vi "NavbalLabVIEW(15-5-28.vi"() -> ()   [LabVIEW 2012] (continued)
              n343 = Index Array(array=w4186, index=1) -> (element=w4183:i32)
              n344 = Insert Into Array(array=w4184, index (dim 1)=w4183, new element=w4182) -> (w4178:dbl[][][])  [unwired: 2 in]
              n345 = Array Size(array=w4178) -> (size(s)=w4180:i32[])
              n346 = Index Array(array=w4180, index=1) -> (element=w4179:i32)
              n347 = Insert Into Array(array=w4178, index (dim 1)=w4179, new element=w4177) -> (w4176:dbl[][][])  [unwired: 2 in]
            }
            frame "LA Class" {
              n348 = Array Size(array=w4200) -> (size(s)=w4201:i32[])
              n349 = Array Size(array=w4203) -> (size(s)=w4206:i32[])
              n350 = Index Array(array=w4201, index=1) -> (element=w4199:i32)
              n351 = Index Array(array=w4206, index=1) -> (element=w4204:i32)
              n352 = Insert Into Array(array=w4200, index (dim 1)=w4199, new element=w4198) -> (w4193:dbl[][][])  [unwired: 2 in]
              n353 = Insert Into Array(array=w4203, index (dim 1)=w4204, new element=w4207) -> (w4194:dbl[][][])  [unwired: 2 in]
              n354 = Array Size(array=w4194) -> (size(s)=w4197:i32[])
              n355 = Index Array(array=w4197, index=1) -> (element=w4195:i32)
              n356 = Insert Into Array(array=w4194, index (dim 1)=w4195, new element=w4193) -> (w4192:dbl[][][])  [unwired: 2 in]
            }
            frame "Ohio Class" {
              n357 = Array Size(array=w4216) -> (size(s)=w4217:i32[])
              n358 = Array Size(array=w4219) -> (size(s)=w4222:i32[])
              n359 = Index Array(array=w4217, index=1) -> (element=w4215:i32)
              n360 = Index Array(array=w4222, index=1) -> (element=w4220:i32)
              n361 = Insert Into Array(array=w4219, index (dim 1)=w4220, new element=w4223) -> (w4210:dbl[][][])  [unwired: 2 in]
              n362 = Insert Into Array(array=w4216, index (dim 1)=w4215, new element=w4214) -> (w4209:dbl[][][])  [unwired: 2 in]
              n363 = Array Size(array=w4210) -> (size(s)=w4213:i32[])
              n364 = Index Array(array=w4213, index=1) -> (element=w4211:i32)
              n365 = Insert Into Array(array=w4210, index (dim 1)=w4211, new element=w4209) -> (w4208:dbl[][][])  [unwired: 2 in]
            }
          }
          n366 = Array Size(array=w3330) -> (size(s)=w3436:i32[])
          n367 = Array Size(array=w3333) -> (size(s)=w3427:i32[])
          n368 = Array Size(array=w3332) -> (size(s)=w3425:i32[])
          n369 = Array Size(array=w3331) -> (size(s)=w3420:i32[])
          n370 = Index Array(array=w3436, index=0) -> (element=w3418:i32)
          n371 = Index Array(array=w3427, index=0) -> (element=w3426:i32)
          n372 = Index Array(array=w3425, index=0) -> (element=w3423:i32)
          n373 = Index Array(array=w3420, index=0) -> (element=w3419:i32)
          n374 = Greater?(x=w3418, y=700) -> (0:w3429:bool)
          n375 = Or(x="Mark Current", y=w3366) -> (x .or. y?=w3367:bool)
          n376 = case shown="True" "Averaging" {
            tunnel: [10 "Number of Averages"] -> w3416
            frame False {
            }
            frame True {
            }
          }
          n377 = case shown="\"Simulated Signals Ohio\"" w3369 {
            tunnel: [w4382 w4431 w4480] -> w3480
            tunnel: [w4386 w4435 w4484] -> w3478
            tunnel: [w4384 w4433 w4482] -> w3523
            tunnel: [w4373 w4428 w4477] -> w3328
            tunnel: [w4385 w4434 w4483] -> w3407
            tunnel: [w4383 w4432 w4481] -> w3406
            tunnel: [w4381 w4430 w4479] -> w3456
            tunnel: [w4380 w4429 w4478] -> w3532
            tunnel: w3530 -> [w4387 w4436 w4485]
            tunnel: w3416 -> [w4374 w4422 w4471]
            frame "Simulated Signals Ohio" {
              # "Ensure that buffer is full before processing"
              # ">>  data out from buffer  >>"
              n378 = local read "Number of Samples"() -> (w4388:i32)
              n379 = call "Convert to Dynamic Data11"("Array"=bool[] [FALSE, FALSE, FALSE, FALSE, FALSE, FALSE, FALSE, FALSE, FALSE, FALSE, TRUE, FALSE, FALSE, FALSE, FALSE, FALSE, FALSE, FALSE, FALSE, FALSE]) -> ("Dynamic Data Type"=w4376:dynamicdata)  [unwired: 3 in]
              n380 = call-poly <userlib>:"Circular Buffer.vi"("Buffer Size"=w4387, "Read Size"=w4388, "Operation"=Circular_Buffer_Operations."Read (most recent)") -> ("Data Out"=w4375:waveform(dbl)[])  [unwired: 5 in, 3 out]
              n381 = call "Select Tach Port2"("Selector Input"=w4376, "Signals"=w4375) -> ("Signal Out"=w4380:dynamicdata)  [unwired: 8 in, 1 out]
              n382 = call "Convert from Dynamic Data49"("Dynamic Data Type"=w4375) -> ("Array"=w4391:dbl[][])  [unwired: 3 in]
              n383 = call "Convert to Dynamic Data10"("Array"=bool[] [TRUE, FALSE, FALSE, FALSE, FALSE, FALSE, FALSE, FALSE, FALSE, FALSE, FALSE, FALSE, FALSE, FALSE, FALSE, FALSE, FALSE, FALSE, FALSE, FALSE]) -> ("Dynamic Data Type"=w4378:dynamicdata)  [unwired: 3 in]
              n384 = Array Size(array=w4391) -> (size(s)=w4394:i32[])
              n385 = call "Select Tach Stbd3"("Selector Input"=w4378, "Signals"=w4375) -> ("Signal Out"=w4373:dynamicdata)  [unwired: 8 in, 1 out]
              n386 = Equal?(x=w4394, y=w4388) -> (x = y?=w4392:bool[])
              n387 = Index Array(array=w4392, index=1) -> (element=w4389:bool)
              n388 = case shown="True" w4389 {
                tunnel: w4375 -> [_ w4414]
                tunnel: [w4395 w4407] -> w4386
                tunnel: [w4397 w4404] -> w4385
                tunnel: [w4395 w4406] -> w4384
                tunnel: [w4395 w4405] -> w4382
                tunnel: [w4397 w4401] -> w4383
                tunnel: [w4397 w4402] -> w4381
                tunnel: w4374 -> [_ w4400]
                frame False {
                  w4395 = cluster{"x0":dbl, "dx":dbl, "magnitude":dbl[]}[] [] ("spectra")
                  n389 = local read "DAQ Start"() -> (w4396:bool)
                  n390 = case shown="True" w4396 {
                    frame False {
                      n391 = property on="DAQ Start" class="Bool (strict)"("BoolText.Text"="DAQ START" ("Boolean Text.Text")) -> ()  [unwired: 2 in, 2 out]
                    }
                    frame True {
                      n392 = property on="DAQ Start" class="Bool (strict)"("BoolText.Text"="Buffering..." ("Boolean Text.Text")) -> ()  [unwired: 2 in, 2 out]
                    }
                  }
                  n393 = local read "Default Stbd Graph"() -> (w4397:dynamicdata)
                }
                frame True {
                  # "convert to VdB"
                  # "convert to VdB"
                  # "convert to VdB"
                  n394 = local read "DAQ Start"() -> (w4403:bool)
                  n395 = case shown="True" w4403 {
                    frame False {
                    }
                    frame True {
                      n396 = property on="DAQ Start" class="Bool (strict)"("BoolText.Text"="DAQ STOP" ("Boolean Text.Text")) -> ()  [unwired: 2 in, 2 out]
                    }
                  }
                  n397 = call "Convert to Dynamic Data3"("Array"=bool[] [FALSE, FALSE, FALSE, FALSE, FALSE, FALSE, FALSE, FALSE, FALSE, FALSE, TRUE, TRUE, TRUE, TRUE, TRUE, TRUE, TRUE, TRUE, TRUE, TRUE]) -> ("Dynamic Data Type"=w4415:dynamicdata)  [unwired: 3 in]
                  n398 = call "Select Port"("Selector Input"=w4415, "Signals"=w4414) -> ("Signal Out"=w4401:dynamicdata)  [unwired: 8 in, 1 out]
                  n399 = call "Convert to Dynamic Data2"("Array"=bool[] [TRUE, TRUE, TRUE, TRUE, TRUE, TRUE, TRUE, TRUE, TRUE, TRUE, FALSE, FALSE, FALSE, FALSE, FALSE, FALSE, FALSE, FALSE, FALSE, FALSE]) -> ("Dynamic Data Type"=w4419:dynamicdata)  [unwired: 3 in]
                  n400 = call "Select Stbd"("Selector Input"=w4419, "Signals"=w4414) -> ("Signal Out"=w4404:dynamicdata)  [unwired: 8 in, 1 out]
                  n401 = call "Convert to Dynamic Data4"("Array"=bool[] [FALSE, FALSE, FALSE, FALSE, FALSE, FALSE, FALSE, FALSE, FALSE, FALSE, FALSE, FALSE, FALSE, FALSE, FALSE, FALSE, FALSE, FALSE, FALSE, FALSE, TRUE, TRUE, TRUE, TRUE, TRUE, TRUE, TRUE, TRUE, TRUE, TRUE, TRUE, TRUE]) -> ("Dynamic Data Type"=w4416:dynamicdata)  [unwired: 3 in]
                  n402 = call "Select Corner"("Selector Input"=w4416, "Signals"=w4414) -> ("Signal Out"=w4402:dynamicdata)  [unwired: 8 in, 1 out]
                  n403 = call-poly <vilib>:"SVL Set dB Reference.vi"("dB reference [EU]"=3.937e-07, "scaled signals in [EU]"=w4404) -> ("scaled signals out [EU]"=w4412:waveform(dbl)[])  [unwired: 8 in, 1 out]
                  n404 = call-poly <vilib>:"SVL Set dB Reference.vi"("dB reference [EU]"=3.937e-07, "scaled signals in [EU]"=w4402) -> ("scaled signals out [EU]"=w4408:waveform(dbl)[])  [unwired: 8 in, 1 out]
                  n405 = call-poly <vilib>:"SVL Set dB Reference.vi"("dB reference [EU]"=3.937e-07, "scaled signals in [EU]"=w4401) -> ("scaled signals out [EU]"=w4410:waveform(dbl)[])  [unwired: 8 in, 1 out]
                  n406 = call "Power Spectrum3"("input signals"=w4410, "number of averages"=w4400) -> ("spectra"=w4406:cluster{"x0":dbl, "dx":dbl, "magnitude":dbl[]}[])  [unwired: 12 in, 5 out]
                  n407 = call "Power Spectrum6"("input signals"=w4408, "number of averages"=w4400) -> ("spectra"=w4405:cluster{"x0":dbl, "dx":dbl, "magnitude":dbl[]}[])  [unwired: 12 in, 5 out]
                  n408 = call "Power Spectrum2"("input signals"=w4412, "number of averages"=w4400) -> ("spectra"=w4407:cluster{"x0":dbl, "dx":dbl, "magnitude":dbl[]}[])  [unwired: 12 in, 5 out]
                }
              }
            }
            frame "LA Class" {
              # "Ensure that buffer is full before processing"
              # ">>  data out from buffer  >>"
              n409 = local read "Number of Samples"() -> (w4437:i32)
              n410 = call "Convert to Dynamic Data19"("Array"=bool[] [FALSE, FALSE, FALSE, FALSE, FALSE, FALSE, FALSE, FALSE, FALSE, FALSE, FALSE, FALSE, FALSE, FALSE, FALSE, FALSE, FALSE, FALSE, FALSE, FALSE, FALSE, FALSE, FALSE, FALSE, FALSE, TRUE]) -> ("Dynamic Data Type"=w4424:dynamicdata)  [unwired: 3 in]
              n411 = call-poly <userlib>:"Circular Buffer.vi"("Buffer Size"=w4436, "Read Size"=w4437, "Operation"=Circular_Buffer_Operations."Read (most recent)") -> ("Data Out"=w4423:waveform(dbl)[])  [unwired: 5 in, 3 out]
              n412 = call "Select Tach Port4"("Selector Input"=w4424, "Signals"=w4423) -> ("Signal Out"=w4429:dynamicdata)  [unwired: 8 in, 1 out]
              n413 = call "Convert from Dynamic Data5"("Dynamic Data Type"=w4423) -> ("Array"=w4440:dbl[][])  [unwired: 3 in]
              n414 = call "Convert to Dynamic Data18"("Array"=bool[] [TRUE, FALSE, FALSE, FALSE, FALSE, FALSE, FALSE, FALSE, FALSE, FALSE, FALSE, FALSE, FALSE, FALSE, FALSE, FALSE, FALSE, FALSE, FALSE, FALSE]) -> ("Dynamic Data Type"=w4426:dynamicdata)  [unwired: 3 in]
              n415 = Array Size(array=w4440) -> (size(s)=w4443:i32[])
              n416 = call "Select Tach Stbd2"("Selector Input"=w4426, "Signals"=w4423) -> ("Signal Out"=w4428:dynamicdata)  [unwired: 8 in, 1 out]
              n417 = Equal?(x=w4443, y=w4437) -> (x = y?=w4441:bool[])
              n418 = Index Array(array=w4441, index=1) -> (element=w4438:bool)
              n419 = case shown="False" w4438 {
                tunnel: w4423 -> [_ w4466]
                tunnel: [w4444 w4459] -> w4435
                tunnel: [w4446 w4456] -> w4434
                tunnel: [w4444 w4458] -> w4433
                tunnel: [w4444 w4457] -> w4431
                tunnel: [w4446 w4453] -> w4432
                tunnel: [w4446 w4454] -> w4430
                tunnel: w4422 -> [_ w4452]
                frame False {
                  w4444 = cluster{"x0":dbl, "dx":dbl, "magnitude":dbl[]}[] [] ("spectra")
                  n420 = local read "DAQ Start"() -> (w4445:bool)
                  n421 = case shown="True" w4445 {
                    frame False {
                      n422 = property on="DAQ Start" class="Bool (strict)"("BoolText.Text"="DAQ START" ("Boolean Text.Text")) -> ()  [unwired: 2 in, 2 out]
                    }
                    frame True {
                      n423 = property on="DAQ Start" class="Bool (strict)"("BoolText.Text"="Buffering..." ("Boolean Text.Text")) -> ()  [unwired: 2 in, 2 out]
                    }
                  }
                  n424 = local read "Default Stbd Graph"() -> (w4446:dynamicdata)
                }
                frame True {
                  # "convert to VdB"
                  # "convert to VdB"
                  # "convert to VdB"
                  n425 = local read "DAQ Start"() -> (w4455:bool)
                  n426 = case shown="True" w4455 {
                    frame False {
                    }
                    frame True {
                      n427 = property on="DAQ Start" class="Bool (strict)"("BoolText.Text"="DAQ STOP" ("Boolean Text.Text")) -> ()  [unwired: 2 in, 2 out]
                    }
                  }
                  n428 = call "Convert to Dynamic Data16"("Array"=bool[] [FALSE, FALSE, FALSE, FALSE, FALSE, FALSE, FALSE, FALSE, FALSE, FALSE, FALSE, FALSE, FALSE, FALSE, FALSE, FALSE, FALSE, FALSE, FALSE, FALSE, FALSE, FALSE, FALSE, FALSE, FALSE, TRUE, TRUE, TRUE, TRUE, TRUE, TRUE, TRUE, TRUE, TRUE, TRUE, TRUE, TRUE, TRUE]) -> ("Dynamic Data Type"=w4467:dynamicdata)  [unwired: 3 in]
                  n429 = call "Select Port3"("Selector Input"=w4467, "Signals"=w4466) -> ("Signal Out"=w4453:dynamicdata)  [unwired: 8 in, 1 out]
                  n430 = call "Convert to Dynamic Data15"("Array"=bool[] [TRUE, FALSE, FALSE, FALSE, FALSE, FALSE, FALSE, FALSE, FALSE, FALSE, FALSE, FALSE, FALSE, TRUE, TRUE, TRUE, TRUE, TRUE, TRUE, TRUE, TRUE, TRUE, TRUE, TRUE, TRUE, FALSE, FALSE, FALSE, FALSE, FALSE, FALSE, FALSE, FALSE, FALSE, FALSE, FALSE, FALSE, FALSE]) -> ("Dynamic Data Type"=w4469:dynamicdata)  [unwired: 3 in]
                  n431 = call "Select Stbd4"("Selector Input"=w4469, "Signals"=w4466) -> ("Signal Out"=w4456:dynamicdata)  [unwired: 8 in, 1 out]
                  n432 = call "Convert to Dynamic Data17"("Array"=bool[] [FALSE, TRUE, TRUE, TRUE, TRUE, TRUE, TRUE, TRUE, TRUE, TRUE, TRUE, TRUE, TRUE, FALSE, FALSE, FALSE, FALSE, FALSE, FALSE, FALSE, FALSE, FALSE, FALSE, FALSE, FALSE, FALSE, FALSE, FALSE, FALSE, FALSE, FALSE, FALSE, FALSE, FALSE, FALSE, FALSE, FALSE, FALSE]) -> ("Dynamic Data Type"=w4468:dynamicdata)  [unwired: 3 in]
                  n433 = call "Select Corner4"("Selector Input"=w4468, "Signals"=w4466) -> ("Signal Out"=w4454:dynamicdata)  [unwired: 8 in, 1 out]
                  n434 = call-poly <vilib>:"SVL Set dB Reference.vi"("dB reference [EU]"=3.937e-07, "scaled signals in [EU]"=w4456) -> ("scaled signals out [EU]"=w4464:waveform(dbl)[])  [unwired: 8 in, 1 out]
                  n435 = call-poly <vilib>:"SVL Set dB Reference.vi"("dB reference [EU]"=3.937e-07, "scaled signals in [EU]"=w4454) -> ("scaled signals out [EU]"=w4460:waveform(dbl)[])  [unwired: 8 in, 1 out]
                  n436 = call-poly <vilib>:"SVL Set dB Reference.vi"("dB reference [EU]"=3.937e-07, "scaled signals in [EU]"=w4453) -> ("scaled signals out [EU]"=w4462:waveform(dbl)[])  [unwired: 8 in, 1 out]
                  n437 = call "Power Spectrum12"("input signals"=w4460, "number of averages"=w4452) -> ("spectra"=w4457:cluster{"x0":dbl, "dx":dbl, "magnitude":dbl[]}[])  [unwired: 12 in, 5 out]
                  n438 = call "Power Spectrum11"("input signals"=w4462, "number of averages"=w4452) -> ("spectra"=w4458:cluster{"x0":dbl, "dx":dbl, "magnitude":dbl[]}[])  [unwired: 12 in, 5 out]
                  n439 = call "Power Spectrum10"("input signals"=w4464, "number of averages"=w4452) -> ("spectra"=w4459:cluster{"x0":dbl, "dx":dbl, "magnitude":dbl[]}[])  [unwired: 12 in, 5 out]
                }
              }
            }
            frame "Ohio Class" {
              # "Ensure that buffer is full before processing"
              # ">>  data out from buffer  >>"
              n440 = local read "Number of Samples"() -> (w4486:i32)
              n441 = call "Convert to Dynamic Data24"("Array"=bool[] [FALSE, FALSE, FALSE, FALSE, FALSE, FALSE, FALSE, FALSE, FALSE, FALSE, FALSE, FALSE, FALSE, FALSE, FALSE, FALSE, FALSE, FALSE, FALSE, FALSE, FALSE, FALSE, TRUE]) -> ("Dynamic Data Type"=w4473:dynamicdata)  [unwired: 3 in]
              n442 = call-poly <userlib>:"Circular Buffer.vi"("Buffer Size"=w4485, "Read Size"=w4486, "Operation"=Circular_Buffer_Operations."Read (most recent)") -> ("Data Out"=w4472:waveform(dbl)[])  [unwired: 5 in, 3 out]
              n443 = call "Select Tach Port5"("Selector Input"=w4473, "Signals"=w4472) -> ("Signal Out"=w4478:dynamicdata)  [unwired: 8 in, 1 out]
              n444 = call "Convert from Dynamic Data6"("Dynamic Data Type"=w4472) -> ("Array"=w4489:dbl[][])  [unwired: 3 in]
              n445 = call "Convert to Dynamic Data23"("Array"=bool[] [TRUE, FALSE, FALSE, FALSE, FALSE, FALSE, FALSE, FALSE, FALSE, FALSE, FALSE, FALSE, FALSE, FALSE, FALSE, FALSE, FALSE, FALSE, FALSE, FALSE]) -> ("Dynamic Data Type"=w4475:dynamicdata)  [unwired: 3 in]
              n446 = Array Size(array=w4489) -> (size(s)=w4492:i32[])
              n447 = call "Select Tach Stbd5"("Selector Input"=w4475, "Signals"=w4472) -> ("Signal Out"=w4477:dynamicdata)  [unwired: 8 in, 1 out]
              n448 = Equal?(x=w4492, y=w4486) -> (x = y?=w4490:bool[])
              n449 = Index Array(array=w4490, index=1) -> (element=w4487:bool)
              n450 = case shown="False" w4487 {
                tunnel: w4472 -> [_ w4512]
                tunnel: [w4493 w4505] -> w4484
                tunnel: [w4495 w4502] -> w4483
                tunnel: [w4493 w4504] -> w4482
                tunnel: [w4493 w4503] -> w4480
                tunnel: [w4495 w4499] -> w4481
                tunnel: [w4495 w4500] -> w4479
                tunnel: w4471 -> [_ w4498]
                frame False {
                  w4493 = cluster{"x0":dbl, "dx":dbl, "magnitude":dbl[]}[] [] ("spectra")
                  n451 = local read "DAQ Start"() -> (w4494:bool)
                  n452 = case shown="True" w4494 {
                    frame False {
                      n453 = property on="DAQ Start" class="Bool (strict)"("BoolText.Text"="DAQ START" ("Boolean Text.Text")) -> ()  [unwired: 2 in, 2 out]
                    }
                    frame True {
                      n454 = property on="DAQ Start" class="Bool (strict)"("BoolText.Text"="Buffering..." ("Boolean Text.Text")) -> ()  [unwired: 2 in, 2 out]
                    }
                  }
                  n455 = local read "Default Stbd Graph"() -> (w4495:dynamicdata)
                }
                frame True {
                  # "convert to VdB"
                  # "convert to VdB"
                  # "convert to VdB"
                  n456 = local read "DAQ Start"() -> (w4501:bool)
                  n457 = case shown="True" w4501 {
                    frame False {
                    }
                    frame True {
                      n458 = property on="DAQ Start" class="Bool (strict)"("BoolText.Text"="DAQ STOP" ("Boolean Text.Text")) -> ()  [unwired: 2 in, 2 out]
                    }
                  }
                  n459 = call "Convert to Dynamic Data21"("Array"=bool[] [FALSE, FALSE, FALSE, FALSE, FALSE, FALSE, FALSE, FALSE, FALSE, FALSE, FALSE, FALSE, FALSE, FALSE, FALSE, FALSE, FALSE, FALSE, FALSE, FALSE, FALSE, FALSE, TRUE, TRUE, TRUE, TRUE, TRUE, TRUE, TRUE, TRUE, TRUE, TRUE]) -> ("Dynamic Data Type"=w4513:dynamicdata)  [unwired: 3 in]
                  n460 = call "Select Port5"("Selector Input"=w4513, "Signals"=w4512) -> ("Signal Out"=w4499:dynamicdata)  [unwired: 8 in, 1 out]
                  n461 = call "Convert to Dynamic Data20"("Array"=bool[] [TRUE, FALSE, FALSE, FALSE, FALSE, FALSE, FALSE, FALSE, FALSE, FALSE, FALSE, FALSE, FALSE, TRUE, TRUE, TRUE, TRUE, TRUE, TRUE, TRUE, TRUE, TRUE]) -> ("Dynamic Data Type"=w4517:dynamicdata)  [unwired: 3 in]
                  n462 = call "Select Stbd5"("Selector Input"=w4517, "Signals"=w4512) -> ("Signal Out"=w4502:dynamicdata)  [unwired: 8 in, 1 out]
                  n463 = call "Convert to Dynamic Data22"("Array"=bool[] [FALSE, TRUE, TRUE, TRUE, TRUE, TRUE, TRUE, TRUE, TRUE, TRUE, TRUE, TRUE, TRUE, FALSE, FALSE, FALSE, FALSE, FALSE, FALSE, FALSE, FALSE, FALSE, FALSE, FALSE, FALSE, FALSE, FALSE, FALSE, FALSE, FALSE, FALSE, FALSE]) -> ("Dynamic Data Type"=w4514:dynamicdata)  [unwired: 3 in]
                  n464 = call "Select Corner5"("Selector Input"=w4514, "Signals"=w4512) -> ("Signal Out"=w4500:dynamicdata)  [unwired: 8 in, 1 out]
                  n465 = call-poly <vilib>:"SVL Set dB Reference.vi"("dB reference [EU]"=3.937e-07, "scaled signals in [EU]"=w4502) -> ("scaled signals out [EU]"=w4510:waveform(dbl)[])  [unwired: 8 in, 1 out]
                  n466 = call-poly <vilib>:"SVL Set dB Reference.vi"("dB reference [EU]"=3.937e-07, "scaled signals in [EU]"=w4500) -> ("scaled signals out [EU]"=w4506:waveform(dbl)[])  [unwired: 8 in, 1 out]
                  n467 = call-poly <vilib>:"SVL Set dB Reference.vi"("dB reference [EU]"=3.937e-07, "scaled signals in [EU]"=w4499) -> ("scaled signals out [EU]"=w4508:waveform(dbl)[])  [unwired: 8 in, 1 out]
                  n468 = call "Power Spectrum15"("input signals"=w4506, "number of averages"=w4498) -> ("spectra"=w4503:cluster{"x0":dbl, "dx":dbl, "magnitude":dbl[]}[])  [unwired: 12 in, 5 out]
                  n469 = call "Power Spectrum13"("input signals"=w4510, "number of averages"=w4498) -> ("spectra"=w4505:cluster{"x0":dbl, "dx":dbl, "magnitude":dbl[]}[])  [unwired: 12 in, 5 out]
                  n470 = call "Power Spectrum14"("input signals"=w4508, "number of averages"=w4498) -> ("spectra"=w4504:cluster{"x0":dbl, "dx":dbl, "magnitude":dbl[]}[])  [unwired: 12 in, 5 out]
                }
              }
            }
          }
          "Default Stbd Graph" <- w3407
          "spectra" <- w3523
          n471 = call "Convert from Dynamic Data48"("Dynamic Data Type"=w3532) -> ("Array"=w3544:dbl[])  [unwired: 3 in]
          n472 = Array Max & Min(array=w3544) -> (max value=w3533:dbl)  [unwired: 3 out]
          n473 = Greater?(x=w3533, y=1.0) -> (0:w3542:bool)
          n474 = case shown="True" w3542 {
            tunnel: w3532 -> [_ w4362]
            tunnel: [0.0 ("detected frequency") w4359] -> w3538
            frame False {
            }
            frame True {
              n475 = call "Filter2"("Lower Cut-Off"="Port Tach Cutoff Freq", "Signal"=w4362) -> ("Filtered Signal"=w4357:dynamicdata)  [unwired: 8 in, 1 out]
              n476 = call "Power Spectrum4"("input signals"=w4357) -> ("spectra"=→"Port Tach Spectra":cluster{"x0":dbl, "dx":dbl, "magnitude":dbl[]}[])  [unwired: 13 in, 5 out]
              n477 = call-poly <vilib>:"Extract Single Tone Information.vi"("time signals in"=w4357) -> ("detected frequencies"=w4361:dbl[])  [unwired: 5 in, 5 out]
              n478 = Index Array(array=w4361, index=0) -> (element=w4359:dbl)
            }
          }
          "Frequency (Hz) 2" <- w3538
          n479 = Multiply(x=w3538, y=60.0) -> (x*y=→"Frequency (RPM) 2":dbl)
          n480 = In Range and Coerce(upper limit=60.6, x=w3538, lower limit=60.4) -> (In Range?=w3535:bool)  [unwired: 1 out]
          n481 = case shown="True" w3535 {
            tunnel: [u32 16752008 u32 5308226] -> w3534
            frame False {
            }
            frame True {
            }
          }
          n482 = property on="Frequency (Hz) 2" class="DigNum (strict)"("NumText.BGColor"=w3534) -> ()  [unwired: 2 in, 2 out]
          n483 = property on="Frequency (RPM) 2" class="DigNum (strict)"("NumText.BGColor"=w3534) -> ()  [unwired: 2 in, 2 out]
          n484 = call "Convert from Dynamic Data47"("Dynamic Data Type"=w3328) -> ("Array"=w3554:dbl[])  [unwired: 3 in]
          n485 = Array Max & Min(array=w3554) -> (max value=w3551:dbl)  [unwired: 3 out]
          n486 = Greater?(x=w3551, y=1.0) -> (0:w3552:bool)
          n487 = case shown="True" w3552 {
            tunnel: w3328 -> [_ w4370]
            tunnel: [0.0 ("detected frequency") w4369] -> w3537
            frame False {
            }
            frame True {
              n488 = call "Filter"("Lower Cut-Off"="Stbd Tach Cutoff Freq", "Signal"=w4370) -> ("Filtered Signal"=w4367:dynamicdata)  [unwired: 8 in, 1 out]
              n489 = call-poly <vilib>:"Extract Single Tone Information.vi"("time signals in"=w4367) -> ("detected frequencies"=w4371:dbl[])  [unwired: 5 in, 5 out]
              n490 = Index Array(array=w4371, index=0) -> (element=w4369:dbl)
              n491 = call "Power Spectrum"("input signals"=w4367) -> ("spectra"=→"Starboard Tach Spectra":cluster{"x0":dbl, "dx":dbl, "magnitude":dbl[]}[])  [unwired: 13 in, 5 out]
            }
          }
          "Frequency (Hz) 1" <- w3537
          n492 = Multiply(x=w3537, y=60.0) -> (x*y=→"Frequency (RPM) 1":dbl)
          n493 = In Range and Coerce(upper limit=59.6, x=w3537, lower limit=59.4) -> (In Range?=w3549:bool)  [unwired: 1 out]
          n494 = case shown="True" w3549 {
            tunnel: [u32 16752008 u32 5308226] -> w3545
            frame False {
            }
            frame True {
            }
          }
          n495 = property on="Frequency (Hz) 1" class="DigNum (strict)"("NumText.BGColor"=w3545) -> ()  [unwired: 2 in, 2 out]
          n496 = property on="Frequency (RPM) 1" class="DigNum (strict)"("NumText.BGColor"=w3545) -> ()  [unwired: 2 in, 2 out]
          n497 = case shown="True" w3367 {
            frame False {
            }
            frame True {
              n498 = local read "time string"() -> (→"Marker Time":string)
              n499 = local read "Mils/Sec-Phase(CORNERS-Stbd)"() -> (w4242:sgl[][])
              n500 = local read "Mils/Sec-Phase(CORNERS-Port)"() -> (w4245:sgl[][])
              n501 = local read "Mils/Sec-Phase(STBD)"() -> (w4244:dbl[][])
              n502 = local read "Mils/Sec-Phase(PORT)"() -> (w4243:sgl[][])
              n503 = Array Size(array=w4242) -> (size(s)=w4241:i32[])
              n504 = Index Array(array=w4241, index=0) -> (element=w4239:i32)
              n505 = Insert Into Array(array=w4242, index (row)=w4239, new element #1=w4245, new element #2=w4244, new element #3=w4243) -> (w4238:sgl[][])  [unwired: 1 in]
              n506 = local read "Marker Mag"() -> (w4234:sgl[][])
              n507 = local read "Marker Phase"() -> (w4227:sgl[][])
              n508 = Index Array "Mag"(array=w4238, index (col)=0 ("disabled index (col)")) -> (element=w4235:sgl[])  [unwired: 1 in]
              n509 = Index Array "Phase"(array=w4238, index (col)=1 ("disabled index (col)")) -> (element=w4226:sgl[])  [unwired: 1 in]
              n510 = Array Size(array=w4234) -> (size(s)=w4233:i32[])
              n511 = Array Size(array=w4227) -> (size(s)=w4228:i32[])
              n512 = Index Array(array=w4233, index=1) -> (element=w4231:i32)
              n513 = Insert Into Array(array=w4234, index (col)=w4231, new element=w4235) -> (→"Marker Mag":sgl[][])  [unwired: 1 in]
              n514 = Index Array(array=w4228, index=1) -> (element=w4225:i32)
              n515 = Insert Into Array(array=w4227, index (col)=w4225, new element=w4226) -> (→"Marker Phase":sgl[][])  [unwired: 1 in]
            }
          }
          n516 = case shown="True" w3429 {
            tunnel: [w3940 w3944] -> w3434
            tunnel: w3333 -> [w3940 w3957]
            tunnel: [w3939 w3943] -> w3433
            tunnel: w3332 -> [w3939 w3955]
            tunnel: [w3938 w3942] -> w3432
            tunnel: w3331 -> [w3938 w3950]
            tunnel: [w3937 w3941] -> w3431
            tunnel: w3330 -> [w3937 w3948]
            tunnel: w3426 -> [_ w3956]
            tunnel: w3423 -> [_ w3954]
            tunnel: 600 ("y") -> [_ w3945]
            tunnel: w3419 -> [_ w3951]
            tunnel: w3418 -> [_ w3947]
            frame False {
            }
            frame True {
              n517 = Subtract(x=w3956, y=w3945) -> (x-y=w3953:i32)
              n518 = Subtract(x=w3954, y=w3945) -> (x-y=w3952:i32)
              n519 = Subtract(x=w3951, y=w3945) -> (x-y=w3949:i32)
              n520 = Subtract(x=w3947, y=w3945) -> (x-y=w3946:i32)
              n521 = Delete From Array(array=w3957, length=w3953, index (dim 0)=w3945) -> (array with subset deleted=w3944:dbl[][][])  [unwired: 2 in, 1 out]
              n522 = Delete From Array(array=w3955, length=w3952, index (dim 0)=w3945) -> (array with subset deleted=w3943:dbl[][][])  [unwired: 2 in, 1 out]
              n523 = Delete From Array(array=w3950, length=w3949, index (dim 0)=w3945) -> (array with subset deleted=w3942:dbl[][][])  [unwired: 2 in, 1 out]
              n524 = Delete From Array(array=w3948, length=w3946, index (dim 0)=w3945) -> (array with subset deleted=w3941:dbl[][][])  [unwired: 2 in, 1 out]
            }
          }
          n525 = Array Subset(array=w3334, index (dim 0)=0 ("index"), length (dim 0)=600 ("length"), index (dim 1)="DAQ Listbox", length (dim 1)=1 ("length"), index (dim 2)=0 ("index"), length (dim 2)=2 ("length")) -> (w3610:dbl[][][])
          n526 = Array Subset(array=w3334, index (dim 0)=0 ("index"), length (dim 0)=1 ("length"), index (dim 1)="DAQ Listbox", length (dim 1)=1 ("length"), index (dim 2)=0 ("index"), length (dim 2)=2 ("length")) -> (w3595:dbl[][][])
          n527 = Reshape Array(w3610, 600 ("dimension size"), 2 ("dimension size")) -> (w3572:dbl[][])
          n528 = Reshape Array(w3595, 1 ("dimension size"), 2 ("dimension size")) -> (w3582:dbl[][])
          n529 = Index Array(array=w3582, index (col)=0 ("disabled index (col)")) -> (element=w3584:dbl[])  [unwired: 1 in]
          n530 = Index Array(array=w3582, index (col)=1 ("disabled index (col)")) -> (element=w3581:dbl[])  [unwired: 1 in]
          n531 = Array Subset(array=w3572, index (row)=0 ("index"), length (row)=600 ("length"), index (col)=0 ("index"), length (col)=1 ("length")) -> (w3573:dbl[][])
          n532 = Array Subset(array=w3572, index (row)=0 ("index"), length (row)=600 ("length"), index (col)=1 ("index"), length (col)=1 ("length")) -> (w3597:dbl[][])
          n533 = Reshape Array(w3584, 1 ("dimension size")) -> (w3585:dbl[])
          n534 = Reshape Array(w3581, 1 ("dimension size")) -> (w3591:dbl[])
          n535 = Index Array(array=w3585, index=0) -> (element=w3579:dbl)
          n536 = Index Array(array=w3591, index=0) -> (element=w3616:dbl)
          n537 = Reshape Array(w3597, 600 ("dimension size")) -> (w3576:dbl[])
          n538 = Reshape Array(w3573, 600 ("dimension size")) -> (w3580:dbl[])
          n539 = Insert Into Array(array=w3580, index=0, new element=w3579) -> (→"mag":dbl[])
          n540 = Insert Into Array(array=w3576, index=0, new element=w3616) -> (→"phase":dbl[])
          n541 = property on="Tab 3" class="TabCtl (strict)"() -> ("Visible"=w3443:bool)  [unwired: 2 in, 2 out]
          n542 = property on="Tab 3" class="TabCtl (strict)"() -> ("Value"=w3446:T9)  [unwired: 2 in, 2 out]
          n543 = Equal?(x=w3446, y=T19."Step 6: Polar Plots") -> (x = y?=w3444:bool)
          n544 = And(x=w3444, y=w3443) -> (x .and. y?=w3442:bool)
          n545 = case shown="True" w3442 {
            frame False {
            }
            frame True {
              w3989 = 0 ("index")
              w4002 = T21."Application Font" ("desired font(Application)")
              w4004 = cluster{"width":i16, "height":i16} {"width"=575, "height"=575} ("dimensions (w,h)")
              # "Find the max magnitude to be plotted,\nand adjust the scaling of all plots"
              # "Add Corresponding Prediction measurement to Polar plot"
              # "Add Corresponding Baseline measurement to Polar plot"
              # "Polar Plot"
              n546 = local read "Marker Phase"() -> (w3970:sgl[][])
              n547 = local read "Pred plot"() -> (w3958:dbl[][])
              n548 = local read "Marker Mag"() -> (w3963:sgl[][])
              n549 = Array Size(array=w3963) -> (size(s)=w3966:i32[])
              n550 = local read "Ref Pt Plot"() -> (w3976:sgl[][])
              n551 = Index Array(array=w3966, index=1) -> (element=w3964:i32)
              n552 = local read "DAQ Listbox"() -> (w3969:i32)
              n553 = Index Array(array=w3958, index (col)=1 ("disabled index (col)")) -> (element=w3959:dbl[])  [unwired: 1 in]
              n554 = Index Array(array=w3958, index (col)=0 ("disabled index (col)")) -> (element=w3960:dbl[])  [unwired: 1 in]
              n555 = for {
                N: w3964 -> [_]
                tunnel: [w4013] -> w3968
                tunnel: [w4015] -> w3967 mode=indexing
                tunnel: w3969 -> [w4014]
                tunnel: w3970 -> [w4008]
                tunnel: w3963 -> [w4007]
                i -> [w4011]
                n556 = Index Array(array=w4007, index (row)=w4014) -> (element=w4013:sgl[])  [unwired: 1 in]
                n557 = Index Array(array=w4008, index (row)=w4014) -> (element=w4012:sgl[])  [unwired: 1 in]
                n558 = Index Array(array=w4012, index=w4011) -> (element=w4009:sgl)
                n559 = Index Array(array=w4013, index=w4011) -> (element=w4010:sgl)
                n560 = Bundle(w4010, w4009) -> (w4015:cluster{sgl, sgl})  [unwired: 1 in]
              }
              n561 = Index Array(array=w3976, index (col)=0 ("disabled index (col)")) -> (element=w3978:sgl[])  [unwired: 1 in]
              n562 = Index Array(array=w3976, index (col)=1 ("disabled index (col)")) -> (element=w3975:sgl[])  [unwired: 1 in]
              n563 = Index Array(array=w3959, index=w3969) -> (element=w3991:dbl)
              n564 = Index Array(array=w3960, index=w3969) -> (element=w3988:dbl)
              n565 = for {
                N: 600 -> [_]
                tunnel: [w4020] -> w4003 mode=indexing
                i -> [w4021]
                n566 = local read "phase"() -> (w4016:dbl[])
                n567 = local read "mag"() -> (w4017:dbl[])
                n568 = Index Array(array=w4017, index=w4021) -> (element=w4019:dbl)
                n569 = Index Array(array=w4016, index=w4021) -> (element=w4018:dbl)
                n570 = Bundle("mag. (Vpeak)"=w4019, "mag. (Vpeak)"=w4018) -> (w4020:cluster{"mag. (Vpeak)":dbl, "mag. (Vpeak)":dbl})  [unwired: 1 in]
              }
              n571 = local read "mag"() -> (w3994:dbl[])
              n572 = Bundle("Real Matrix Element"=w3988, "Real Matrix Element"=w3991) -> (w3983:T22)  [unwired: 1 in]
              n573 = Index Array(array=w3978, index=w3969) -> (element=w3993:sgl)
              n574 = Index Array(array=w3975, index=w3969) -> (element=w3997:sgl)
              n575 = Insert Into Array(array=w3994, index=w3989, new element #1=w3993, new element #2=0 ("new element/subarray"), new element #3=w3968) -> (w3990:dbl[])
              n576 = Bundle(w3993, w3997) -> (w3996:cluster{sgl, sgl})  [unwired: 1 in]
              n577 = Initialize Array(w3983, 1 ("dimension size")) -> (w3982:T23)
              n578 = Initialize Array(w3996, 1 ("dimension size")) -> (w3992:cluster{sgl, sgl}[])
              n579 = Insert Into Array(array=w3990, index=w3989, new element=w3988) -> (w3987:dbl[])
              n580 = Array Max & Min(array=w3987) -> (max value=w3980:dbl)  [unwired: 3 out]
              n581 = Divide(x=w3980, y=0.9) -> (x/y=w3971:dbl)
              n582 = property on="maximum" class="DigNum (strict)"("Val(Sgnl)"=w3971) -> ()  [unwired: 2 in, 2 out]
              n583 = call <vilib>:"Polar Plot(points&line).vi"("polar attributes"="polar attributes", "desired font(Application)"=w4002, "dimensions (w,h)"=w4004, "data array [mag, phase (deg)]"=w4003) -> ("new picture"=w3999:picture)  [unwired: 7 in]
              n584 = property on="maximum" class="DigNum (strict)"("Val(Sgnl)"=w3971) -> ()  [unwired: 2 in, 2 out]
              n585 = property on="maximum" class="DigNum (strict)"("Val(Sgnl)"=w3971) -> ()  [unwired: 2 in, 2 out]
              n586 = property on="maximum" class="DigNum (strict)"("Val(Sgnl)"=w3971) -> ()  [unwired: 2 in, 2 out]
              n587 = feedback #1() -> (w3998:picture)  [unwired: 1 in]
              n588 = call <vilib>:"Polar Plot(points&line).vi"("polar attributes"="polar attributes Prediction", "desired font(Application)"=w4002, "dimensions (w,h)"=w4004, "data array [mag, phase (deg)]"=w3982, "picture"=w3998) -> ("new picture"=w3986:picture)  [unwired: 6 in]
              n589 = call <vilib>:"Polar Plot(points&line).vi"("polar attributes"="polar attributes Start Point", "desired font(Application)"=w4002, "dimensions (w,h)"=w4004, "data array [mag, phase (deg)]"=w3992, "picture"=w3986) -> ("new picture"=w3973:picture)  [unwired: 6 in]
              n590 = call <vilib>:"Polar Plot(points&line).vi"("polar attributes"="polar attributes Marker", "desired font(Application)"=w4002, "dimensions (w,h)"=w4004, "data array [mag, phase (deg)]"=w3967, "picture"=w3973) -> ("new picture"=→"Polar Plot Picture":picture)  [unwired: 6 in]
              n591 = feedback-in #1(w3999) -> ()
            }
          }
          n592 = local read "Ship Class"() -> (w3555:T4)
          n593 = local read "Frequency (Hz) 1"() -> (w3556:dbl)
          n594 = case shown="\"LA Class\"" w3555 {
            tunnel: w3407 -> [w4860 w4875 w4876]
            tunnel: [w4846 w4861 w4878] -> w3457
            tunnel: [w4859 w4874 w4877] -> w3477
            frame "LA Class" {
              n595 = Split Signals(w4860) -> (w4859:dynamicdata, w4858:dynamicdata, w4857:dynamicdata, w4856:dynamicdata, w4855:dynamicdata, w4854:dynamicdata, w4853:dynamicdata, w4852:dynamicdata, w4851:dynamicdata, w4850:dynamicdata, w4849:dynamicdata, w4848:dynamicdata, w4847:dynamicdata)  [unwired: 13 in]
              n596 = Merge Signals(w4858, w4857, w4856, w4855, w4854, w4853, w4852, w4851, w4850, w4849, w4848, w4847) -> (w4846:dynamicdata)
            }
            frame "Ohio Class" {
              n597 = Split Signals(w4875) -> (w4874:dynamicdata, w4873:dynamicdata, w4872:dynamicdata, w4871:dynamicdata, w4870:dynamicdata, w4869:dynamicdata, w4868:dynamicdata, w4867:dynamicdata, w4866:dynamicdata, w4865:dynamicdata, w4864:dynamicdata, w4863:dynamicdata, w4862:dynamicdata)  [unwired: 13 in]
              n598 = Merge Signals(w4873, w4872, w4871, w4870, w4869, w4868, w4867, w4866, w4865, w4864, w4863, w4862) -> (w4861:dynamicdata)
            }
            frame "Simulated Signals Ohio" {
              n599 = Split Signals(w4876) -> (w4877:dynamicdata, w4879:dynamicdata, w4880:dynamicdata, w4881:dynamicdata, w4882:dynamicdata, w4883:dynamicdata, w4884:dynamicdata, w4885:dynamicdata, w4886:dynamicdata, w4887:dynamicdata)  [unwired: 10 in]
              n600 = Merge Signals(w4879, w4880, w4881, w4882, w4883, w4884, w4885, w4886, w4887) -> (w4878:dynamicdata)
            }
          }
          n601 = local read "Sample Frequency (Hz)"() -> (w3528:i32)
          n602 = local read "Sample Frequency (Hz)"() -> (w3529:i32)
          n603 = local read "Sample Frequency (Hz)"() -> (w3527:i32)
          n604 = local read "Sample Frequency (Hz)"() -> (w3482:i32)
          n605 = case shown="\"Simulated Signals Ohio\"" w3555 {
            tunnel: w3406 -> [w4807 w4830 w4845]
            tunnel: [w4806 w4816 w4831] -> w3665
            tunnel: [w4805 w4829 w4844] -> w3666
            frame "Simulated Signals Ohio" {
              n606 = Split Signals(w4807) -> (w4805:dynamicdata, w4808:dynamicdata, w4809:dynamicdata, w4810:dynamicdata, w4811:dynamicdata, w4812:dynamicdata, w4813:dynamicdata, w4814:dynamicdata, w4815:dynamicdata, w4804:dynamicdata)  [unwired: 10 in]
              n607 = Merge Signals(w4808, w4809, w4810, w4811, w4812, w4813, w4814, w4815, w4804) -> (w4806:dynamicdata)
            }
            frame "LA Class" {
              n608 = Split Signals(w4830) -> (w4829:dynamicdata, w4828:dynamicdata, w4827:dynamicdata, w4826:dynamicdata, w4825:dynamicdata, w4824:dynamicdata, w4823:dynamicdata, w4822:dynamicdata, w4821:dynamicdata, w4820:dynamicdata, w4819:dynamicdata, w4818:dynamicdata, w4817:dynamicdata)  [unwired: 13 in]
              n609 = Merge Signals(w4828, w4827, w4826, w4825, w4824, w4823, w4822, w4821, w4820, w4819, w4818, w4817) -> (w4816:dynamicdata)
            }
            frame "Ohio Class" {
              n610 = Split Signals(w4845) -> (w4844:dynamicdata, w4843:dynamicdata, w4842:dynamicdata, w4841:dynamicdata, w4840:dynamicdata, w4839:dynamicdata, w4838:dynamicdata, w4837:dynamicdata, w4836:dynamicdata, w4835:dynamicdata, w4834:dynamicdata, w4833:dynamicdata, w4832:dynamicdata)  [unwired: 13 in]
              n611 = Merge Signals(w4843, w4842, w4841, w4840, w4839, w4838, w4837, w4836, w4835, w4834, w4833, w4832) -> (w4831:dynamicdata)
            }
          }
          n612 = local read "Frequency (Hz) 2"() -> (w3557:dbl)
          n613 = local read "Frequency (Hz) 1"() -> (w3643:dbl)
          n614 = local read "Frequency (Hz) 2"() -> (w3483:dbl)
          n615 = Array Size(array=w3523) -> (size(s)=w3520:i32)
          n616 = Array Size(array=w3478) -> (size(s)=w3531:i32)
          n617 = Decrement(x=w3520) -> (x-1=w3519:i32)
          n618 = Decrement(x=w3531) -> (x-1=w3521:i32)
          n619 = Array Size(array=w3480) -> (size(s)=w3571:i32)
          n620 = Array Size(array=w3480) -> (size(s)=w3481:i32)
          n621 = for "Phase (Degrees)" {
            N: w3519 -> [_]
            tunnel: w3406 -> [w4983]
            tunnel: [w4985] -> w3691 mode=indexing
            tunnel: w3528 -> [w4984]
            i -> [w4988]
            n622 = Add(x=1, y=w4988) -> (x+y=w4986:i32)
            n623 = call "Convert from Dynamic Data30"("Dynamic Data Type"=w4983, "Channel"=w4986) -> ("Array"=w4991:dbl[])  [unwired: 2 in]
            n624 = call "Convert from Dynamic Data31"("Dynamic Data Type"=w4983, "Channel"=0) -> ("Array"=w4989:dbl[])  [unwired: 2 in]
            n625 = Reciprocal(x=w4984) -> (1/x=w4995:dbl)
            n626 = call <vilib>:"Cross Power Spectrum.vi"("dt"=w4995, "Signal Y (V)"=w4991, "Signal X (V)"=w4989) -> ("Cross Power XY Spectrum Phase (radians)"=w4982:dbl[])  [unwired: 2 out]
            n627 = Divide(x=180, y=3.141592653589793) -> (x/y=w4992:dbl)
            n628 = Multiply(x=w4982, y=w4992) -> (x*y=w4985:dbl[])
          }
          n629 = for "Magnitude (VdB)" {
            N: w3521 -> [_]
            tunnel: w3478 -> [w5057]
            tunnel: [w5053] -> w3704 mode=indexing
            i -> [w5056]
            n630 = Add(x=1, y=w5056) -> (x+y=w5054:i32)
            n631 = Index Array(array=w5057, index=w5054) -> (element=w5058:cluster{"x0":dbl, "dx":dbl, "magnitude":dbl[]})
            n632 = Unbundle(w5058) -> ("magnitude"=w5053:dbl[])  [unwired: 2 out]
          }
          n633 = Index Array(array=w3478) -> (element=w3705:cluster{"x0":dbl, "dx":dbl, "magnitude":dbl[]})  [unwired: 1 in]
          n634 = for "Phase (Degrees)" {
            N: w3521 -> [_]
            tunnel: w3407 -> [w5095]
            tunnel: [w5091] -> w3559 mode=indexing
            tunnel: w3529 -> [w5089]
            i -> [w5093]
            n635 = Add(x=1, y=w5093) -> (x+y=w5090:i32)
            n636 = call "Convert from Dynamic Data27"("Dynamic Data Type"=w5095, "Channel"=w5090) -> ("Array"=w5097:dbl[])  [unwired: 2 in]
            n637 = call "Convert from Dynamic Data28"("Dynamic Data Type"=w5095, "Channel"=0) -> ("Array"=w5094:dbl[])  [unwired: 2 in]
            n638 = Reciprocal(x=w5089) -> (1/x=w5102:dbl)
            n639 = call <vilib>:"Cross Power Spectrum.vi"("dt"=w5102, "Signal Y (V)"=w5097, "Signal X (V)"=w5094) -> ("Cross Power XY Spectrum Phase (radians)"=w5101:dbl[])  [unwired: 2 out]
            n640 = Divide(x=180, y=3.141592653589793) -> (x/y=w5098:dbl)
            n641 = Multiply(x=w5101, y=w5098) -> (x*y=w5091:dbl[])
          }
          n642 = for "Magnitude (VdB)" {
            N: w3519 -> [_]
            tunnel: w3523 -> [w4949]
            tunnel: [w4945] -> w3689 mode=indexing
            i -> [w4948]
            n643 = Add(x=1, y=w4948) -> (x+y=w4946:i32)
            n644 = Index Array(array=w4949, index=w4946) -> (element=w4950:cluster{"x0":dbl, "dx":dbl, "magnitude":dbl[]})
            n645 = Unbundle(w4950) -> ("magnitude"=w4945:dbl[])  [unwired: 2 out]
          }
          n646 = Index Array(array=w3523) -> (element=w3690:cluster{"x0":dbl, "dx":dbl, "magnitude":dbl[]})  [unwired: 1 in]
          n647 = for "Magnitude (VdB)" {
            N: w3571 -> [_]
            tunnel: w3480 -> [w4758]
            tunnel: [w4757] -> w3662 mode=indexing
            i -> [w4756]
            n648 = Index Array(array=w4758, index=w4756) -> (element=w4759:cluster{"x0":dbl, "dx":dbl, "magnitude":dbl[]})
            n649 = Unbundle(w4759) -> ("magnitude"=w4757:dbl[])  [unwired: 2 out]
          }
          n650 = Unbundle(w3705) -> ("dx"=w3703:dbl)  [unwired: 2 out]
          "frequency resolution" <- w3703
          n651 = Index Array(array=w3480) -> (element=w3663:cluster{"x0":dbl, "dx":dbl, "magnitude":dbl[]})  [unwired: 1 in]
          n652 = for "Phase (Degrees)" {
            N: w3571 -> [_]
            tunnel: w3456 -> [w4796]
            tunnel: [w4794] -> w3664 mode=indexing
            tunnel: w3407 -> [w4792]
            tunnel: w3527 -> [w4791]
            i -> [w4793]
            n653 = call "Convert from Dynamic Data33"("Dynamic Data Type"=w4796, "Channel"=w4793) -> ("Array"=w4798:dbl[])  [unwired: 2 in]
            n654 = call "Convert from Dynamic Data34"("Dynamic Data Type"=w4792, "Channel"=0) -> ("Array"=w4795:dbl[])  [unwired: 2 in]
            n655 = Reciprocal(x=w4791) -> (1/x=w4803:dbl)
            n656 = call <vilib>:"Cross Power Spectrum.vi"("dt"=w4803, "Signal Y (V)"=w4798, "Signal X (V)"=w4795) -> ("Cross Power XY Spectrum Phase (radians)"=w4802:dbl[])  [unwired: 2 out]
            n657 = Divide(x=180, y=3.141592653589793) -> (x/y=w4799:dbl)
            n658 = Multiply(x=w4802, y=w4799) -> (x*y=w4794:dbl[])
          }
          n659 = Unbundle(w3690) -> ("dx"=w3688:dbl)  [unwired: 2 out]
          n660 = for "Magnitude (VdB)" {
            N: w3481 -> [_]
            tunnel: w3480 -> [w4307]
            tunnel: [w4306] -> w3513 mode=indexing
            i -> [w4305]
            n661 = Index Array(array=w4307, index=w4305) -> (element=w4308:cluster{"x0":dbl, "dx":dbl, "magnitude":dbl[]})
            n662 = Unbundle(w4308) -> ("magnitude"=w4306:dbl[])  [unwired: 2 out]
          }
          n663 = Index Array(array=w3480) -> (element=w3514:cluster{"x0":dbl, "dx":dbl, "magnitude":dbl[]})  [unwired: 1 in]
          n664 = for "Phase (Degrees)" {
            N: w3481 -> [_]
            tunnel: w3456 -> [w4345]
            tunnel: [w4343] -> w3515 mode=indexing
            tunnel: w3406 -> [w4341]
            tunnel: w3482 -> [w4340]
            i -> [w4342]
            n665 = call "Convert from Dynamic Data"("Dynamic Data Type"=w4345, "Channel"=w4342) -> ("Array"=w4347:dbl[])  [unwired: 2 in]
            n666 = call "Convert from Dynamic Data2"("Dynamic Data Type"=w4341, "Channel"=0) -> ("Array"=w4344:dbl[])  [unwired: 2 in]
            n667 = Reciprocal(x=w4340) -> (1/x=w4352:dbl)
            n668 = call <vilib>:"Cross Power Spectrum.vi"("dt"=w4352, "Signal Y (V)"=w4347, "Signal X (V)"=w4344) -> ("Cross Power XY Spectrum Phase (radians)"=w4351:dbl[])  [unwired: 2 out]
            n669 = Divide(x=180, y=3.141592653589793) -> (x/y=w4348:dbl)
            n670 = Multiply(x=w4351, y=w4348) -> (x*y=w4343:dbl[])
          }
          n671 = Unbundle(w3663) -> ("dx"=w3661:dbl)  [unwired: 2 out]
          "frequency (resolution) corner" <- w3661
          n672 = Unbundle(w3514) -> ("dx"=w3512:dbl)  [unwired: 2 out]
          "frequency (resolution) corners-port" <- w3512
          n673 = for "Mag (VdB)(8x)" {
            N: w3521 -> [_]
            tunnel: w3704 -> [w5039]
            tunnel: w3703 -> [w5037]
            tunnel: w3556 -> [w5035]
            tunnel: [w5034] -> w3696 mode=indexing
            i -> [w5036]
            n674 = Index Array(array=w5039, index (row)=w5036) -> (element=w5033:dbl[])  [unwired: 1 in]
            n675 = for {
              N: 8 -> [_]
              tunnel: [w5044] -> w5034 mode=indexing
              tunnel: w5033 -> [w5048]
              tunnel: w5035 -> [w5050]
              tunnel: w5037 -> [w5052]
              i -> [w5049]
              w5042 = ext 2.0  # change
              n676 = Divide(x=w5050, y=w5052) -> (x/y=w5040:dbl)
              n677 = Multiply(x=w5040, y=w5049) -> (x*y=w5051:dbl)
              n678 = Add(x=w5040, y=w5051) -> (x+y=w5046:dbl)
              n679 = Subtract(x=w5046, y=w5042) -> (x-y=w5047:ext)
              n680 = Multiply(x=w5042, y=2.0) -> (x*y=w5041:ext)
              n681 = Array Subset(array=w5048, index=w5047, length=w5041) -> (w5045:dbl[])
              n682 = Array Max & Min(array=w5045) -> (max value=w5044:dbl)  [unwired: 3 out]
            }
          }
          "Magnitude VdB Stbd" <- w3696
          n683 = for "Mag (VdB)(8x)" {
            N: w3519 -> [_]
            tunnel: w3689 -> [w4931]
            tunnel: w3688 -> [w4929]
            tunnel: w3557 -> [w4927]
            tunnel: [w4926] -> w3681 mode=indexing
            i -> [w4928]
            n684 = Index Array(array=w4931, index (row)=w4928) -> (element=w4925:dbl[])  [unwired: 1 in]
            n685 = for {
              N: 8 -> [_]
              tunnel: [w4936] -> w4926 mode=indexing
              tunnel: w4925 -> [w4940]
              tunnel: w4927 -> [w4942]
              tunnel: w4929 -> [w4944]
              i -> [w4941]
              w4934 = ext 2.0  # change
              n686 = Divide(x=w4942, y=w4944) -> (x/y=w4932:dbl)
              n687 = Multiply(x=w4932, y=w4941) -> (x*y=w4943:dbl)
              n688 = Add(x=w4932, y=w4943) -> (x+y=w4938:dbl)
              n689 = Subtract(x=w4938, y=w4934) -> (x-y=w4939:ext)
              n690 = Multiply(x=w4934, y=2.0) -> (x*y=w4933:ext)
              n691 = Array Subset(array=w4940, index=w4939, length=w4933) -> (w4937:dbl[])
              n692 = Array Max & Min(array=w4937) -> (max value=w4936:dbl)  [unwired: 3 out]
            }
          }
          "Magnitude VdB Port" <- w3681
          n693 = for "Mag (VdB)(8x)" {
            N: w3571 -> [_]
            tunnel: w3662 -> [w4743]
            tunnel: w3661 -> [w4741]
            tunnel: w3643 -> [w4739]
            tunnel: [w4738] -> w3644 mode=indexing
            i -> [w4740]
            n694 = Index Array(array=w4743, index (row)=w4740) -> (element=w4737:dbl[])  [unwired: 1 in]
            n695 = for {
              N: 8 -> [_]
              tunnel: [w4749] -> w4738 mode=indexing
              tunnel: w4737 -> [w4751]
              tunnel: w4739 -> [w4753]
              tunnel: w4741 -> [w4755]
              i -> [w4752]
              # "Encompass wider span\nto ensure max capture"
              n696 = Divide(x=w4753, y=w4755) -> (x/y=w4747:dbl)
              n697 = Multiply(x=w4747, y=w4752) -> (x*y=w4754:dbl)
              n698 = Add(x=w4747, y=w4754) -> (x+y=w4746:dbl)
              n699 = Subtract(x=w4746, y=1 ("length")) -> (x-y=w4744:dbl)
              n700 = Array Subset(array=w4751, index=w4744, length=3) -> (w4750:dbl[])
              n701 = Array Max & Min(array=w4750) -> (max value=w4749:dbl)  [unwired: 3 out]
            }
          }
          "Magnitude VdB Corner" <- w3644
          n702 = for "Mag (VdB)(8x)" {
            N: w3481 -> [_]
            tunnel: w3513 -> [w4290]
            tunnel: w3512 -> [w4288]
            tunnel: w3483 -> [w4286]
            tunnel: [w4285] -> w3495 mode=indexing
            i -> [w4287]
            n703 = Index Array(array=w4290, index (row)=w4287) -> (element=w4284:dbl[])  [unwired: 1 in]
            n704 = for {
              N: 8 -> [_]
              tunnel: [w4298] -> w4285 mode=indexing
              tunnel: w4284 -> [w4300]
              tunnel: w4286 -> [w4302]
              tunnel: w4288 -> [w4304]
              i -> [w4301]
              n705 = Divide(x=w4302, y=w4304) -> (x/y=w4297:dbl)
              n706 = Multiply(x=w4297, y=w4301) -> (x*y=w4303:dbl)
              n707 = Subtract(x=w4297, y=1.0) -> (x-y=w4295:dbl)
              n708 = Add(x=w4295, y=w4303) -> (x+y=w4292:dbl)
              n709 = Subtract(x=w4292, y=1 ("length")) -> (x-y=w4291:dbl)
              n710 = Array Subset(array=w4300, index=w4291, length=3) -> (w4299:dbl[])
              n711 = Array Max & Min(array=w4299) -> (max value=w4298:dbl)  [unwired: 3 out]
            }
          }
          "Magnitude VdB Corners-Port" <- w3495
          n712 = for "Phase (8x)" {
            N: w3521 -> [_]
            tunnel: w3559 -> [w5065]
            tunnel: [w5061] -> w3558 mode=indexing
            tunnel: w3556 -> [w5060]
            tunnel: w3703 -> [w5059]
            i -> [w5062]
            n713 = Index Array(array=w5065, index (row)=w5062) -> (element=w5063:dbl[])  [unwired: 1 in]
            n714 = for {
              N: 8 -> [_]
              tunnel: [w5071] -> w5061 mode=indexing
              tunnel: w5063 -> [w5073]
              tunnel: w5060 -> [w5069]
              tunnel: w5059 -> [w5068]
              i -> [w5074]
              n715 = Divide(x=w5069, y=w5068) -> (x/y=w5067:dbl)
              n716 = Multiply(x=w5067, y=w5074) -> (x*y=w5075:dbl)
              n717 = Add(x=w5067, y=w5075) -> (x+y=w5072:dbl)
              n718 = Index Array(array=w5073, index=w5072) -> (element=w5066:dbl)
              n719 = case shown="\"navbal\"" "phase data format" {
                tunnel: w5066 -> [w5080 w5083 w5088]
                tunnel: [w5076 w5082 w5088] -> w5071
                frame "0-360" {
                  n720 = Negate(x=w5080) -> (-x=w5078:dbl)
                  n721 = Less Than 0?(x=w5080) -> (x < 0?=w5081:bool)
                  n722 = Add(x=w5078, y=180.0) -> (x+y=w5077:dbl)
                  n723 = Select(t=w5077, s=w5081, f=w5080) -> (s? t:f=w5076:dbl)
                }
                frame "navbal" {
                  n724 = Negate(x=w5083) -> (-x=w5087:dbl)
                  n725 = Less Than 0?(x=w5083) -> (x < 0?=w5086:bool)
                  n726 = Subtract(x=360.0, y=w5083) -> (x-y=w5085:dbl)
                  n727 = Select(t=w5087, s=w5086, f=w5085) -> (s? t:f=w5082:dbl)
                }
                frame "pass through", Default {
                }
              }
            }
          }
          "Phase Stbd" <- w3558
          n728 = local read "phase data format"() -> (w3517:string)
          n729 = for "Phase (8x)" {
            N: w3519 -> [_]
            tunnel: w3691 -> [w4958]
            tunnel: [w4954] -> w3415 mode=indexing
            tunnel: w3557 -> [w4953]
            tunnel: w3688 -> [w4952]
            tunnel: w3517 -> [w4951]
            i -> [w4955]
            n730 = Index Array(array=w4958, index (row)=w4955) -> (element=w4956:dbl[])  [unwired: 1 in]
            n731 = for {
              N: 8 -> [_]
              tunnel: [w4963] -> w4954 mode=indexing
              tunnel: w4956 -> [w4966]
              tunnel: w4953 -> [w4962]
              tunnel: w4952 -> [w4961]
              tunnel: w4951 -> [w4959]
              i -> [w4967]
              n732 = Divide(x=w4962, y=w4961) -> (x/y=w4960:dbl)
              n733 = Multiply(x=w4960, y=w4967) -> (x*y=w4968:dbl)
              n734 = Add(x=w4960, y=w4968) -> (x+y=w4965:dbl)
              n735 = Index Array(array=w4966, index=w4965) -> (element=w4964:dbl)
              n736 = case shown="\"navbal\"" w4959 {
                tunnel: w4964 -> [w4973 w4976 w4981]
                tunnel: [w4969 w4975 w4981] -> w4963
                frame "0-360" {
                  n737 = Negate(x=w4973) -> (-x=w4971:dbl)
                  n738 = Less Than 0?(x=w4973) -> (x < 0?=w4974:bool)
                  n739 = Add(x=w4971, y=180.0) -> (x+y=w4970:dbl)
                  n740 = Select(t=w4970, s=w4974, f=w4973) -> (s? t:f=w4969:dbl)
                }
                frame "navbal" {
                  n741 = Negate(x=w4976) -> (-x=w4980:dbl)
                  n742 = Less Than 0?(x=w4976) -> (x < 0?=w4979:bool)
                  n743 = Subtract(x=360.0, y=w4976) -> (x-y=w4978:dbl)
                  n744 = Select(t=w4980, s=w4979, f=w4978) -> (s? t:f=w4975:dbl)
                }
                frame "pass through", Default {
                }
              }
            }
          }
          "Phase Port" <- w3415
          n745 = local read "Port/Starboard"() -> (w3329:enum32{"Port Side", "Stbd Side"})
          n746 = local read "phase data format"() -> (w3479:string)
          n747 = for "Phase (8x)" {
            N: w3481 -> [_]
            tunnel: w3515 -> [w4316]
            tunnel: [w4312] -> w3486 mode=indexing
            tunnel: w3483 -> [w4311]
            tunnel: w3512 -> [w4310]
            tunnel: w3479 -> [w4309]
            i -> [w4313]
            n748 = Index Array(array=w4316, index (row)=w4313) -> (element=w4314:dbl[])  [unwired: 1 in]
            n749 = for {
              N: 8 -> [_]
              tunnel: [w4321] -> w4312 mode=indexing
              tunnel: w4314 -> [w4324]
              tunnel: w4311 -> [w4320]
              tunnel: w4310 -> [w4319]
              tunnel: w4309 -> [w4318]
              i -> [w4325]
              n750 = Divide(x=w4320, y=w4319) -> (x/y=w4317:dbl)
              n751 = Multiply(x=w4317, y=w4325) -> (x*y=w4326:dbl)
              n752 = Add(x=w4317, y=w4326) -> (x+y=w4323:dbl)
              n753 = Index Array(array=w4324, index=w4323) -> (element=w4322:dbl)
              n754 = case shown="\"navbal\"" w4318 {
                tunnel: w4322 -> [w4331 w4334 w4339]
                tunnel: [w4327 w4333 w4339] -> w4321
                frame "0-360" {
                  n755 = Negate(x=w4331) -> (-x=w4329:dbl)
                  n756 = Less Than 0?(x=w4331) -> (x < 0?=w4332:bool)
                  n757 = Add(x=w4329, y=180.0) -> (x+y=w4328:dbl)
                  n758 = Select(t=w4328, s=w4332, f=w4331) -> (s? t:f=w4327:dbl)
                }
                frame "navbal" {
                  n759 = Negate(x=w4334) -> (-x=w4338:dbl)
                  n760 = Less Than 0?(x=w4334) -> (x < 0?=w4337:bool)
                  n761 = Subtract(x=360.0, y=w4334) -> (x-y=w4336:dbl)
                  n762 = Select(t=w4338, s=w4337, f=w4336) -> (s? t:f=w4333:dbl)
                }
                frame "pass through", Default {
                }
              }
            }
          }
          "Phase Corner 2" <- w3486
          n763 = property on="Boat File" class="Path"() -> ("Value"=w3337:path)  [unwired: 2 in, 2 out]
          n764 = local read "phase data format"() -> (w3516:string)
          n765 = for "Phase (8x)" {
            N: w3571 -> [_]
            tunnel: w3664 -> [w4767]
            tunnel: [w4763] -> w3618 mode=indexing
            tunnel: w3643 -> [w4762]
            tunnel: w3661 -> [w4761]
            tunnel: w3516 -> [w4760]
            i -> [w4764]
            n766 = Index Array(array=w4767, index (row)=w4764) -> (element=w4765:dbl[])  [unwired: 1 in]
            n767 = for {
              N: 8 -> [_]
              tunnel: [w4772] -> w4763 mode=indexing
              tunnel: w4765 -> [w4775]
              tunnel: w4762 -> [w4771]
              tunnel: w4761 -> [w4770]
              tunnel: w4760 -> [w4769]
              i -> [w4776]
              n768 = Divide(x=w4771, y=w4770) -> (x/y=w4768:dbl)
              n769 = Multiply(x=w4768, y=w4776) -> (x*y=w4777:dbl)
              n770 = Add(x=w4768, y=w4777) -> (x+y=w4774:dbl)
              n771 = Index Array(array=w4775, index=w4774) -> (element=w4773:dbl)
              n772 = case shown="\"navbal\"" w4769 {
                tunnel: w4773 -> [w4782 w4785 w4790]
                tunnel: [w4778 w4784 w4790] -> w4772
                frame "0-360" {
                  n773 = Negate(x=w4782) -> (-x=w4780:dbl)
                  n774 = Less Than 0?(x=w4782) -> (x < 0?=w4783:bool)
                  n775 = Add(x=w4780, y=180.0) -> (x+y=w4779:dbl)
                  n776 = Select(t=w4779, s=w4783, f=w4782) -> (s? t:f=w4778:dbl)
                }
                frame "navbal" {
                  n777 = Negate(x=w4785) -> (-x=w4789:dbl)
                  n778 = Less Than 0?(x=w4785) -> (x < 0?=w4788:bool)
                  n779 = Subtract(x=360.0, y=w4785) -> (x-y=w4787:dbl)
                  n780 = Select(t=w4789, s=w4788, f=w4787) -> (s? t:f=w4784:dbl)
                }
                frame "pass through", Default {
